vi "countPath.vi"(2 "inputPath":path, 3 "String":string, 4 "error in (no error)":errorcluster) -> (0 "appended path":path, 1 "error out":errorcluster)   [LabVIEW 2017]
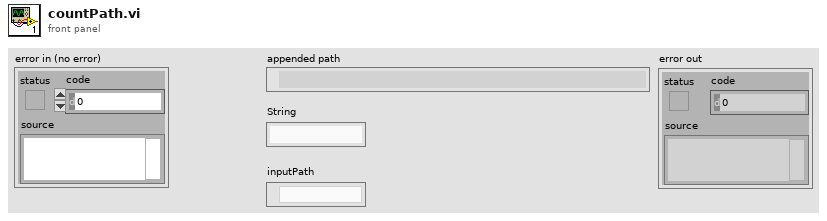
[diagram p1: front panel]
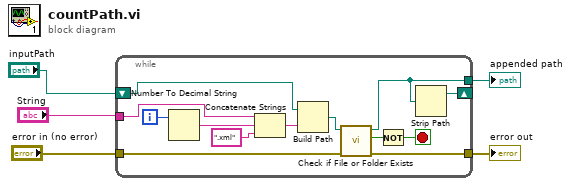
[diagram p0: block diagram]
diagram:
  n1 = while {
    shift-right: [w12] -> _
    shift-left: "inputPath" -> [w13]
    tunnel: [w11] -> w5
    tunnel: "error in (no error)" -> [w8]
    tunnel: [w7] -> w3
    tunnel: "String" -> [w6]
    i -> [w17]
    stop <- w10 stop-if-true
    n2 = Number To Decimal String(number=w17) -> (decimal integer string=w16:string)  [unwired: 1 in]
    n3 = Concatenate Strings(w6, w16, ".xml" ("string")) -> (w15:string)
    n4 = Build Path(base path=w13, name or relative path=w15) -> (appended path=w14:path)
    n5 = call <vilib>:"Check if File or Folder Exists.vi"("error in (no error)"=w8, "path"=w14) -> ("error out"=w7:errorcluster, "file or folder exists?"=w9:bool, "dup path"=w11:path)  [unwired: 7 in]
    n6 = Not(x=w9) -> (.not. x?=w10:bool)
    n7 = Strip Path(path=w11) -> (stripped path=w12:path)  [unwired: 1 out]
  }
  "appended path" <- w5
  "error out" <- w3
